vi "rad deg conversion.vi"(2 "radians":dbl, 3 "degrees":dbl) -> (0 "degrees":dbl, 1 "radians":dbl)   [LabVIEW 2011]
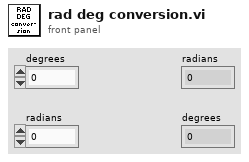
[diagram p1: front panel]
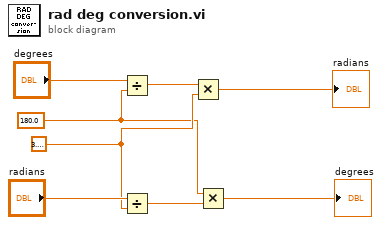
[diagram p0: block diagram]
diagram:
  w2 = 180.0
  w4 = 3.141592653589793
  n1 = Divide(x="degrees", y=w2) -> (x/y=w7:dbl)
  n2 = Divide(x="radians", y=w4) -> (x/y=w3:dbl)
  n3 = Multiply(x=w7, y=w4) -> (x*y=→"radians":dbl)
  n4 = Multiply(x=w2, y=w3) -> (x*y=→"degrees":dbl)
